vi "LoadMap_Interpolation.vi"(9 "Torque":dbl[](array[numeric]) format="%_6g", 10 "Speed_ramp_increment":dbl=1.0, 11 "Speed":dbl[](array[numeric]) format="%_6g") -> (1 "empty?":bool, 2 "Error":bool, 3 "Load_matrix":dbl[][](array[numeric]))   [LabVIEW 2025]
uses:
  <vilib>/Analysis/1siggen.llb/Ramp Pattern by Delta.vi
  <vilib>/gmath/NI_Gmath.lvlib
  <vilib>/Analysis/NI_AALBase.lvlib
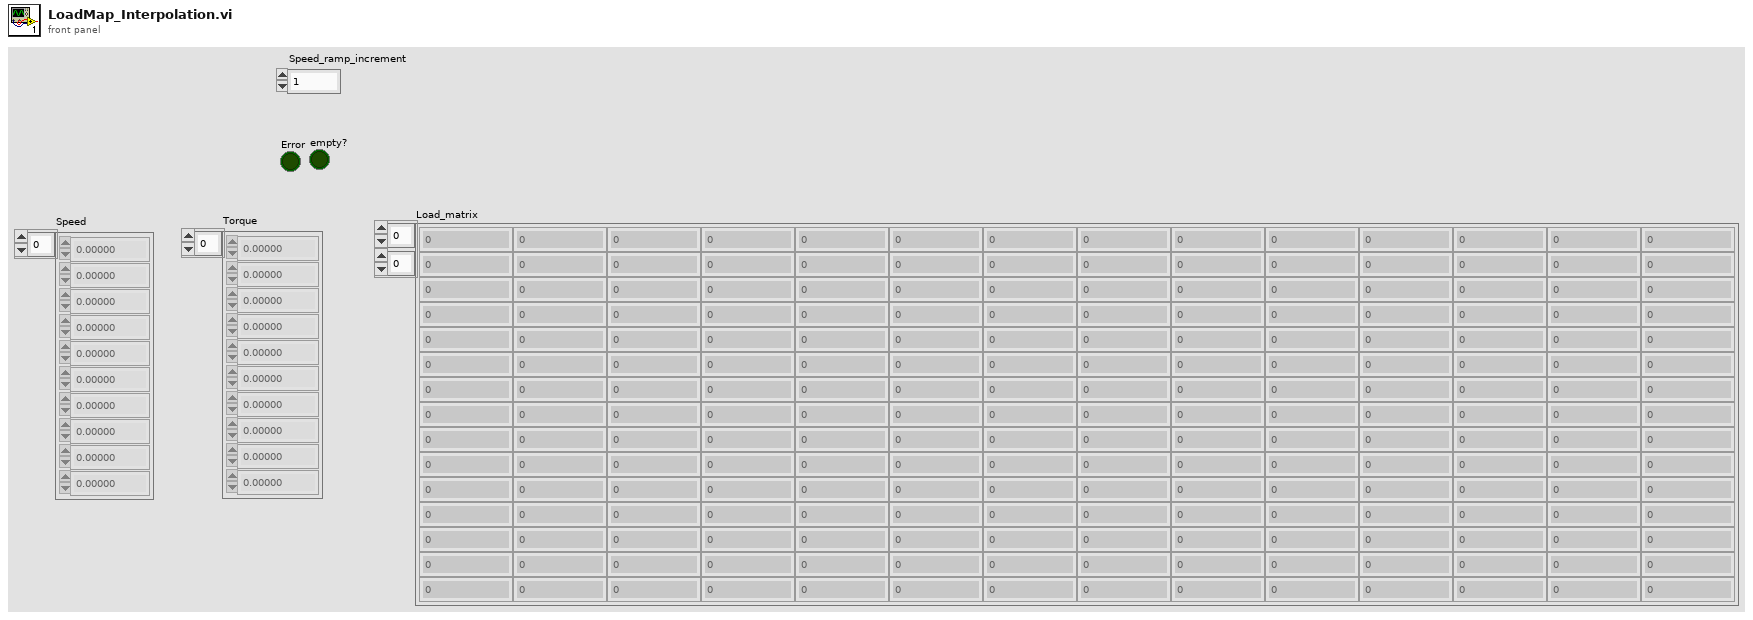
[diagram p1: front panel]
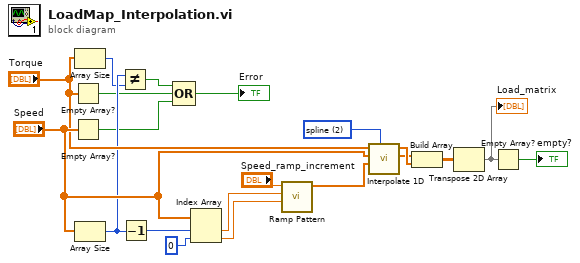
[diagram p0: block diagram]
diagram:
  w16 = 2 items=["nearest", "linear", "spline", "cubic Hermite", "Lagrange"] ("method")
  n1 = Empty Array?(array="Torque") -> (empty?=w5:bool)
  n2 = Empty Array?(array="Speed") -> (empty?=w4:bool)
  n3 = Array Size(array="Torque") -> (size(s)=w7:i32)
  n4 = Array Size(array="Speed") -> (size(s)=w8:i32)
  n5 = Not Equal?(x=w8, y=w7) -> (x != y?=w6:bool)
  n6 = Decrement(x=w8) -> (x-1=w11:i32)
  n7 = Compound Arithmetic op=OR(w6, w5, w4) -> (→"Error":bool)
  n8 = Index Array(array="Speed", index #1=w11, index #2=0 ("index")) -> (element #1=w12:dbl, element #2=w14:dbl)
  n9 = call-poly <vilib>:"Ramp Pattern.vi"("start"=w14, "end"=w12, "delta"="Speed_ramp_increment") -> ("Ramp Pattern"=w20:dbl[])  [unwired: 6 in, 2 out]
  n10 = call <vilib>:"Interpolate 1D.vi"("method"=w16, "xi"=w20, "X"="Speed", "Y"="Torque") -> ("xi used"=w17:dbl[], "yi"=w18:dbl[])  [unwired: 5 in, 1 out]
  n11 = Build Array(w17, w18) -> (w19:dbl[][])
  n12 = Transpose 2D Array(2D array=w19) -> (transposed array=w2:dbl[][])
  "Load_matrix" <- w2
  n13 = Empty Array?(array=w2) -> (empty?=→"empty?":bool)
